vi "Alarma.vi"() -> ()   [LabVIEW 2020]
uses:
  Estados.ctl
panel:
  in  "Temperatura":dbl(slide) scale=0.0..100.0
  in  "stop":bool
  in  "Tiempo(ms)":dbl
  in  "Limite":dbl
  out "Alarma":bool
  out "System":dynamicdata(graph)
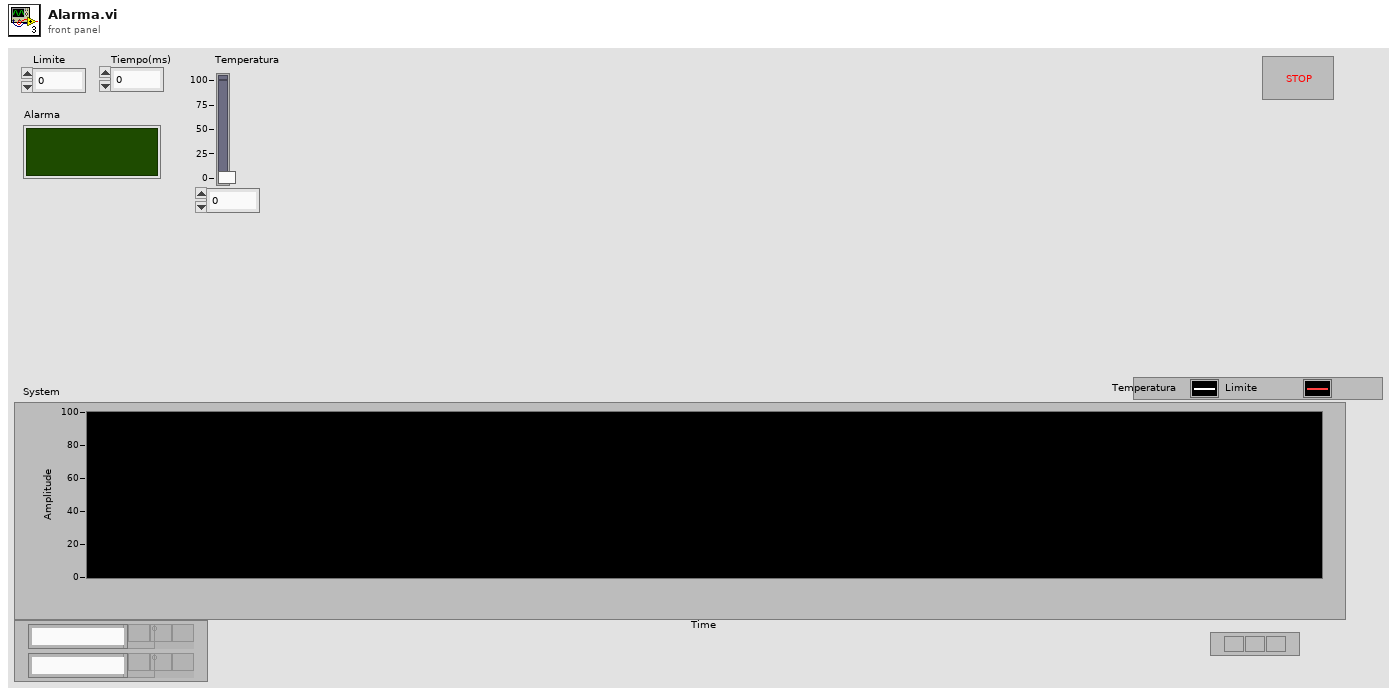
[diagram p1: front panel]
types:
  T1 = typedef "Estados.ctl" = enum16{"Inicio", "Alarma", "DB", "Idle", "DAQ"}
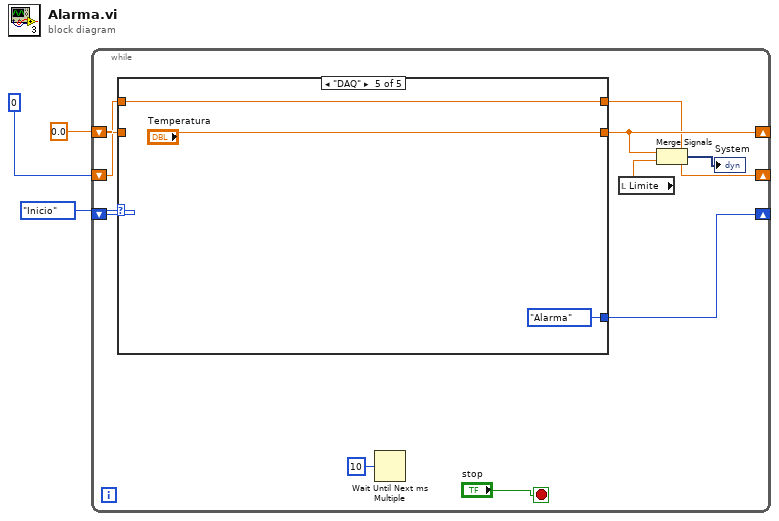
[diagram p0: block diagram]
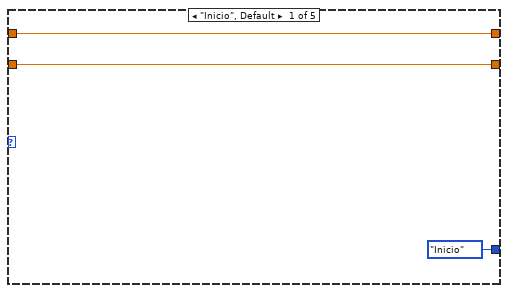
[diagram p2: hidden frame]
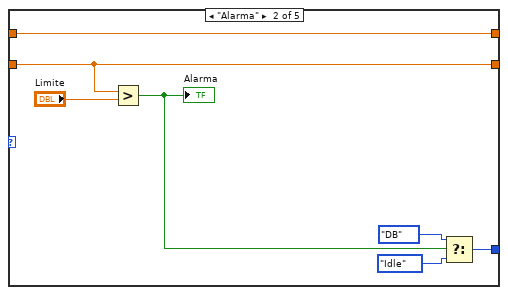
[diagram p3: hidden frame]
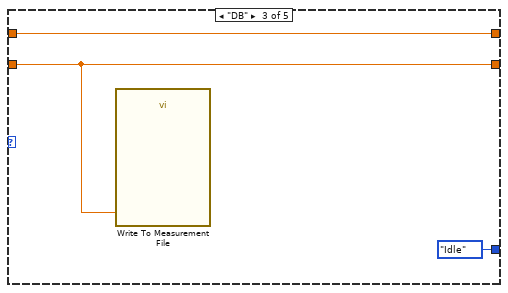
[diagram p4: hidden frame]
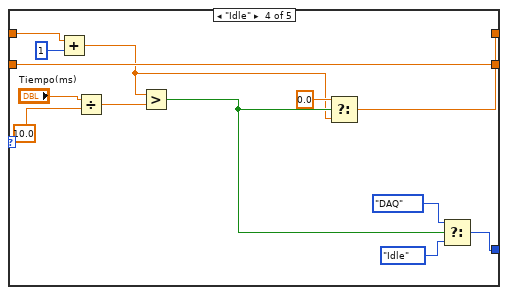
[diagram p5: hidden frame]
diagram:
  n1 = while {
    shift-right: [w10] -> _
    shift-left: Estados."Inicio" ("Estados") -> [w11]
    shift-right: [w8] -> _
    shift-left: 0.0 ("Temperatura") -> [w7]
    shift-right: [w4] -> _
    shift-left: 0 -> [w5]
    stop <- "stop" stop-if-true
    n2 = case shown="\"DAQ\"" w11 {
      tunnel: [Estados."Inicio" ("Estados") w21 Estados."Idle" ("Estados") w31 Estados."Alarma" ("Estados")] -> w10
      tunnel: [w15 w23 w25 w39 "Temperatura"] -> w8
      tunnel: w7 -> [w15 w23 w25 w39 _]
      tunnel: w5 -> [w14 w17 w24 w36 w40]
      tunnel: [w14 w17 w24 w27 w40] -> w4
      frame "Inicio", Default {
      }
      frame "Alarma" {
        n3 = Greater?(x=w23, y="Limite") -> (0:w20:bool)
        "Alarma" <- w20
        n4 = Select(t=Estados."DB" ("Estados"), s=w20, f=Estados."Idle" ("Estados")) -> (s? t:f=w21:T1)
      }
      frame "DB" {
        n5 = call "Write To Measurement File"("Signals"=w25) -> ()  [unwired: 16 in, 3 out]
      }
      frame "Idle" {
        n6 = Add(x=w36, y=1) -> (x+y=w28:dbl)
        n7 = Divide(x="Tiempo(ms)", y=10.0) -> (x/y=w34:dbl)
        n8 = Greater?(x=w28, y=w34) -> (0:w30:bool)
        n9 = Select(t=0.0, s=w30, f=w28) -> (s? t:f=w27:dbl)
        n10 = Select(t=Estados."DAQ" ("Estados"), s=w30, f=Estados."Idle" ("Estados")) -> (s? t:f=w31:T1)
      }
      frame "DAQ" {
      }
    }
    n11 = Wait Until Next ms Multiple(millisecond multiple=u32 10) -> ()  [unwired: 1 out]
    n12 = local read "Limite"() -> (w6:dbl)
    n13 = Merge Signals(w8, w6) -> (→"System":dynamicdata)
  }
